vi "servo.vi"(8 "delay":u32, 9 "in=true\nout = false":bool, 10 "left-right":enum16{"r", "l"}(ring)) -> ()   [LabVIEW 2017]
uses:
  Constant.vi
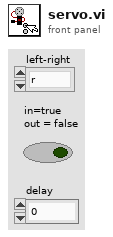
[diagram p1: front panel]
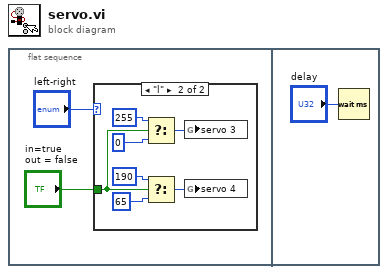
[diagram p0: block diagram]
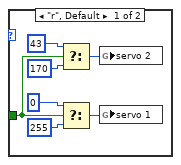
[diagram p2: hidden frame]
diagram:
  n1 = flat-sequence {
    frame #0 {
      n2 = case shown="\"l\"" "left-right" {
        tunnel: "in=true\nout = false" -> [w3 w10]
        frame "r", Default {
          n3 = Select(t=u8 43, s=w3, f=u8 170) -> (s? t:f=w4:u8)
          n4 = Select(t=u8 0, s=w3, f=u8 255) -> (s? t:f=w7:u8)
          n5 = global write "Constant.vi" "servo 2"(w4) -> ()
          n6 = global write "Constant.vi" "servo 1"(w7) -> ()
        }
        frame "l" {
          n7 = Select(t=u8 255, s=w10, f=u8 0) -> (s? t:f=w14:u8)
          n8 = Select(t=u8 190, s=w10, f=u8 65) -> (s? t:f=w11:u8)
          n9 = global write "Constant.vi" "servo 3"(w14) -> ()
          n10 = global write "Constant.vi" "servo 4"(w11) -> ()
        }
      }
    }
    frame #1 {
      n11 = Wait (ms)(milliseconds to wait="delay") -> ()  [unwired: 1 out]
    }
  }
